vi "rszvl Initialize with Options.vi"(0 "VISA resource name":refnum<visa-resource-name>, 2 "Option string (\"\")":string, 5 "ID Query (T: Check)":bool=TRUE, 7 "Reset (T: Reset)":bool=TRUE, 11 "error in (no error)":errorcluster) -> (4 "VISA resource name out":refnum<visa-resource-name>, 15 "error out":errorcluster)   [LabVIEW 2014]
doc: "This VI opens a new session to the instrument.\nCompared to the <b>Initialize.vi</b>, this one allows for additional settings in the <b>Option string</b>."
uses:
  rszvl_core_global.vi
  rszvl_rsidr_core.lvlib
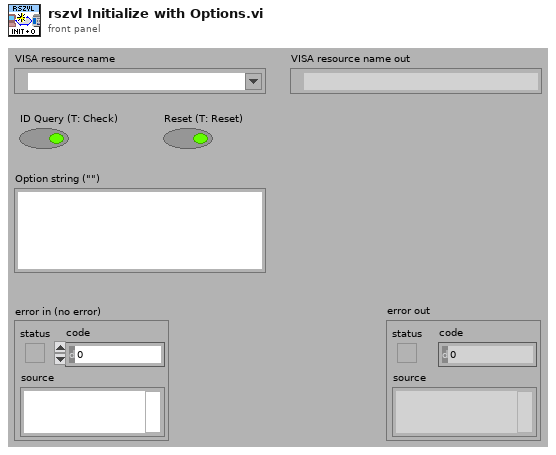
[diagram p1: front panel]
types:
  T1 = cluster{"Level":i32, "Descriptive Name":string, "Class Only":bool, "Data Type":u16, "Access":u16, "Identifier":string, "Range Table":string, "Command":string, "Read Callback":string, "Write Callback":string, "Range Callback":string, "Check Callback":string, "Rngtable Callback":string, "Coerce Callback":string, "User Callback":string, "Supported Models":string, "Instrument Options":string, "Repeated Capabilities":string, "Restricted Repeated Capabilities":string, "Help":string, "Flags":cluster{"OPC Wait":bool, "Dont check status":bool, "*WAI":bool}, "Check Status Callback":string}[]
  T2 = cluster{"repCapName":string, "identifiers":string[], "cmdValues":string[]}[]
  T3 = cluster{"Name":string, "Type":i32, "Min?":bool, "Max?":bool, "Entries":cluster{"Name":string, "Discrete or Min":dbl, "Max":dbl, "Coerced":dbl, "Command":string}[]}[]
  T4 = typedef "rszvl_rsidr_core.lvlib/type_Session_Data.ctl" = cluster{"Instr type":string, "Instr type for err. msg.":string, "Installed Options":string[], "OPC Timeout":i32, "Query Instrument Status":bool, "Check Range":bool, "Check Options":bool, "Add LF to Write":bool, "Simulate":bool, "Logging":bool, "Logging params":variant, "Interface Type":enum16{"Unknown", "GPIB", "VXI", "GPIB_VXI", "ASRL", "PXI", "TCPIP", "USB", "SOCKET"}, "Fast Sweep":i32, "AdditionalFlags":i32, "WaitBeforeWrite":i32, "WaitBeforeRead":i32, "BinDataChunkSize":i64}
  T5 = enum16{"Unknown", "GPIB", "VXI", "GPIB_VXI", "ASRL", "PXI", "TCPIP", "USB", "SOCKET"}
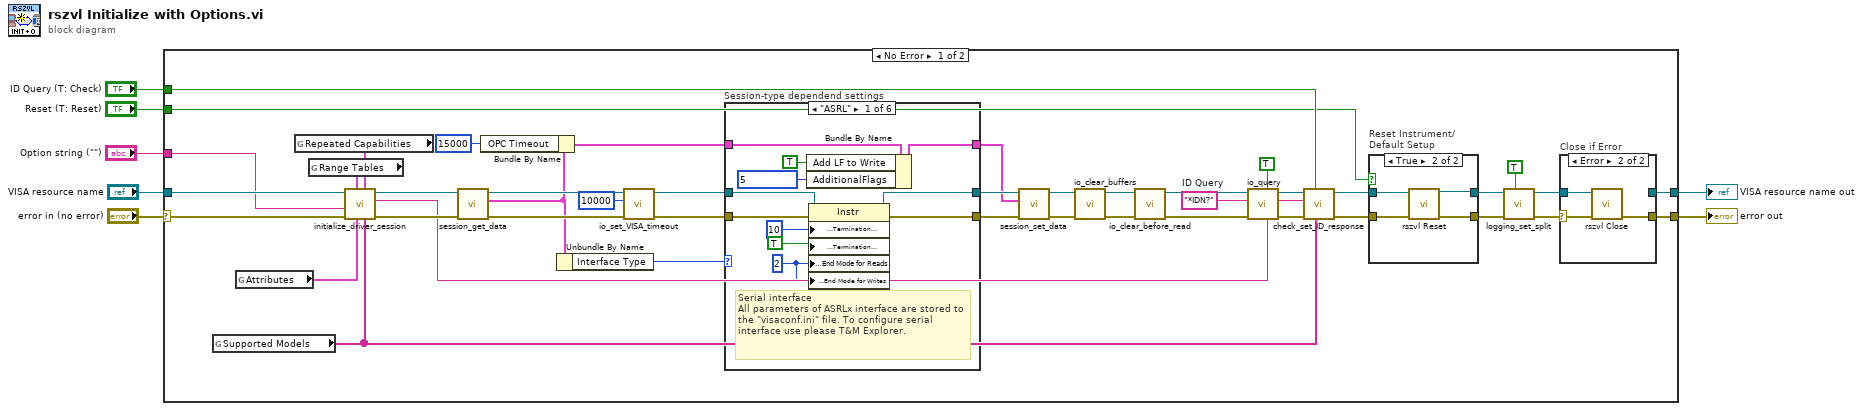
[diagram p0: block diagram]
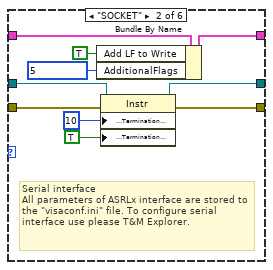
[diagram p2: hidden frame]
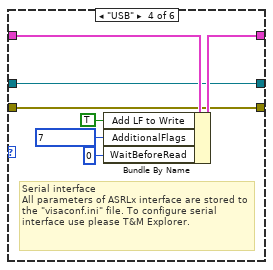
[diagram p4: hidden frame]
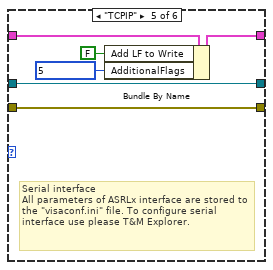
[diagram p5: hidden frame]
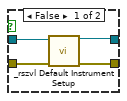
[diagram p8: hidden frame]
diagram:
  n1 = case shown="No Error" "error in (no error)" {
    selector: "error in (no error)" -> [w42 w105]
    tunnel: [w51 _] -> w7
    tunnel: [w43 w105] -> w6
    tunnel: "VISA resource name" -> [w41 _]
    tunnel: "Option string (\"\")" -> [w32 _]
    tunnel: "ID Query (T: Check)" -> [w14 _]
    tunnel: "Reset (T: Reset)" -> [w13 _]
    frame No Error {
      w45 = "*IDN?"  # ID Query
      n2 = global read "rszvl_core_global.vi" "Supported Models"() -> (w11:string[])
      n3 = global read "rszvl_core_global.vi" "Attributes"() -> (w8:T1)
      n4 = global read "rszvl_core_global.vi" "Repeated Capabilities"() -> (w9:T2)
      n5 = global read "rszvl_core_global.vi" "Range Tables"() -> (w10:T3)
      n6 = call "initialize_driver_session.vi"("Supported instruments"=w11, "Repeated Capabilities"=w9, "Attributes"=w8, "Range Tables"=w10, "error in"=w42, "Option String"=w32, "VISA resource name"=w41) -> ("error out"=w35:errorcluster, "Simulation *IDN? response"=w12:string, "VISA resource name out"=w34:refnum<visa-resource-name>)  [unwired: 2 in]
      n7 = call "session_get_data.vi"("error in"=w35, "VISA resource name"=w34) -> ("error out"=w31:errorcluster, "Session User Data out"=w26:T4, "VISA resource name out"=w30:refnum<visa-resource-name>)  [unwired: 7 in]
      n8 = Bundle By Name(cluster=w26, "OPC Timeout"=15000) -> (w28:T4)
      n9 = Unbundle By Name(w26) -> ("Interface Type"=w27:T5)
      n10 = call "io_set_VISA_timeout.vi"("error in"=w31, "VISA Timeout"=u32 10000, "VISA resource name"=w30) -> ("error out"=w22:errorcluster, "VISA resource name out"=w21:refnum<visa-resource-name>)  [unwired: 6 in, 1 out]
      n11 = case "Session-type dependend settings" shown="\"ASRL\"" w27 {
        tunnel: w22 -> [w58 w69 w75 w79 w85 w89]
        tunnel: w21 -> [w59 w70 w74 w78 w84 w90]
        tunnel: [w57 w68 w75 w79 w85 w89] -> w25
        tunnel: [w56 w67 w74 w78 w84 w90] -> w24
        tunnel: w28 -> [w53 w66 w73 w82 w88 w91]
        tunnel: [w52 w65 w73 w81 w87 w91] -> w23
        frame "ASRL" {
          w62 = u16 2 ("ASRL End In")
          # "Serial interface\nAll parameters of ASRLx interface are stored to the \"visaconf.ini\" file. To configure serial interface use please T&M Explorer."
          n12 = Bundle By Name(cluster=w53, "Add LF to Write"=TRUE, "AdditionalFlags"=5) -> (w52:T4)
          n13 = property on="Property Node" class="Instr"(reference=w59, error in=w58, "Message Based Settings:Termination Character"=u8 10 ("TermChar"), "Message Based Settings:Termination Character Enable"=TRUE ("TermChar En"), "Serial Settings:End Mode for Reads"=w62, "Serial Settings:End Mode for Writes"=w62) -> (reference out=w56:refnum<visa-resource-name>, error out=w57:errorcluster)
        }
        frame "SOCKET" {
          # "Serial interface\nAll parameters of ASRLx interface are stored to the \"visaconf.ini\" file. To configure serial interface use please T&M Explorer."
          n14 = Bundle By Name(cluster=w66, "Add LF to Write"=TRUE, "AdditionalFlags"=5) -> (w65:T4)
          n15 = property on="Property Node" class="Instr"(reference=w70, error in=w69, "Message Based Settings:Termination Character"=u8 10 ("TermChar"), "Message Based Settings:Termination Character Enable"=TRUE ("TermChar En")) -> (reference out=w67:refnum<visa-resource-name>, error out=w68:errorcluster)
        }
        frame "GPIB" {
          # "Serial interface\nAll parameters of ASRLx interface are stored to the \"visaconf.ini\" file. To configure serial interface use please T&M Explorer."
        }
        frame "USB" {
          # "Serial interface\nAll parameters of ASRLx interface are stored to the \"visaconf.ini\" file. To configure serial interface use please T&M Explorer."
          n16 = Bundle By Name(cluster=w82, "Add LF to Write"=TRUE, "AdditionalFlags"=7, "WaitBeforeRead"=0 ("WaitBeforeWrite")) -> (w81:T4)
        }
        frame "TCPIP" {
          # "Serial interface\nAll parameters of ASRLx interface are stored to the \"visaconf.ini\" file. To configure serial interface use please T&M Explorer."
          n17 = Bundle By Name(cluster=w88, "Add LF to Write"=FALSE, "AdditionalFlags"=5) -> (w87:T4)
        }
        frame Default {
        }
      }
      n18 = call "session_set_data.vi"("error in"=w25, "Session User Data in"=w23, "VISA resource name"=w24) -> ("error out"=w20:errorcluster, "VISA resource name out"=w19:refnum<visa-resource-name>)  [unwired: 7 in]
      n19 = call "io_clear_buffers.vi"("error in"=w20, "VISA resource name"=w19) -> ("error out"=w18:errorcluster, "VISA resource name out"=w17:refnum<visa-resource-name>)  [unwired: 8 in]
      n20 = call "io_clear_before_read.vi"("error in"=w18, "VISA resource name"=w17) -> ("error out"=w16:errorcluster, "VISA resource name out"=w15:refnum<visa-resource-name>)  [unwired: 8 in]
      n21 = call "io_query.vi"("Simulation read buffer (\"Simulation\")"=w12, "Trim Response (F)"=TRUE, "error in"=w16, "write buffer"=w45, "VISA resource name"=w15) -> ("error out"=w48:errorcluster, "read buffer"=w46:string, "VISA resource name out"=w47:refnum<visa-resource-name>)  [unwired: 3 in, 1 out]
      n22 = call "check_set_ID_response.vi"("Supported instruments in"=w11, "Error if ID Query check fails"=w14, "error in"=w48, "IDN string in"=w46, "VISA resource name"=w47) -> ("error out"=w49:errorcluster, "VISA resource name out"=w50:refnum<visa-resource-name>)  [unwired: 3 in, 2 out]
      n23 = case "Reset Instrument/\nDefault Setup" shown="True" w13 {
        tunnel: w49 -> [w100 w104]
        tunnel: [w99 w103] -> w40
        tunnel: w50 -> [w98 w102]
        tunnel: [w97 w101] -> w39
        frame False {
          n24 = call "_rszvl Default Instrument Setup.vi"("VISA resource name"=w98, "error in (no error)"=w100) -> ("VISA resource name out"=w97:refnum<visa-resource-name>, "error out"=w99:errorcluster)  [unwired: 12 in]
        }
        frame True {
          n25 = call "rszvl Reset.vi"("VISA resource name"=w102, "error in (no error)"=w104) -> ("VISA resource name out"=w101:refnum<visa-resource-name>, "error out"=w103:errorcluster)  [unwired: 12 in]
        }
      }
      n26 = call "logging_set_split.vi"("Evaluate section error (F)"=TRUE, "error in"=w40, "VISA resource name"=w39) -> ("error out"=w38:errorcluster, "VISA resource name out"=w37:refnum<visa-resource-name>)  [unwired: 7 in]
      n27 = case "Close if Error" shown="Error" w38 {
        selector: w38 -> [w92 w95]
        tunnel: w37 -> [w93 w96]
        tunnel: [w93 _] -> w51
        tunnel: [w92 w94] -> w43
        frame No Error {
        }
        frame Error {
          n28 = call "rszvl Close.vi"("error in (no error)"=w95, "VISA resource name"=w96) -> ("error out"=w94:errorcluster)  [unwired: 9 in]
        }
      }
    }
    frame Error {
    }
  }
  "VISA resource name out" <- w7
  "error out" <- w6
